vi "libdaq_gpio_read_bit.vi"(0 "error in (no error)":errorcluster, 1 "device_name":string, 2 "module_name":string, 4 "ioIndex":u8) -> (14 "error out":errorcluster, 15 "device_name":string, 16 "module_name":string, 18 "BitVal":bool=TRUE)   [LabVIEW 2010, in "libdaqVI.lvlib"]
doc: "读取一个输入IO的状态，对一个配置为OUT模式的IO执行读取操作，将会是该IO的输出电压，对一个配置为AF模式的IO执行读取操作，返回结果是不确定的"
uses:
  libdaqVI.lvlib
  dll/daqlib.dll
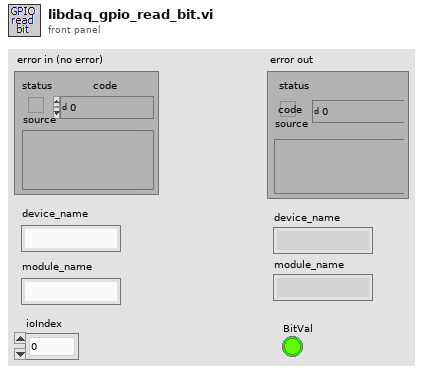
[diagram p1: front panel]
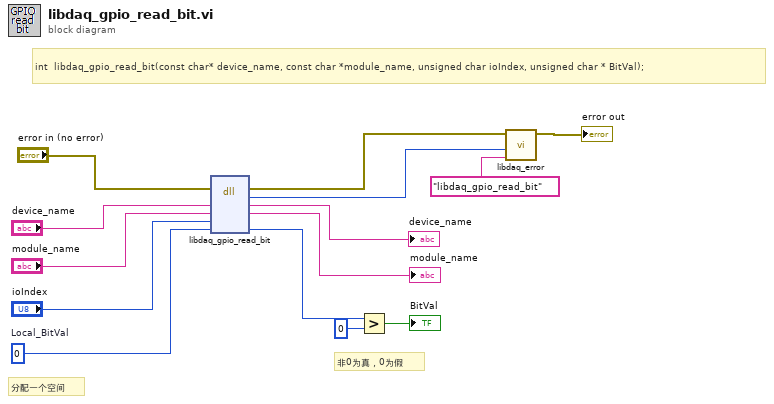
[diagram p0: block diagram]
diagram:
  w4 = u8 0  # Local_BitVal
  # "非0为真，0为假"
  # "分配一个空间"
  # "int  libdaq_gpio_read_bit(const char* device_name, const char *module_name, unsigned char ioIndex, unsigned char * BitVal);"
  n1 = dll-call lib="E:/Product/Example/DAQ-USB3212/Labview/labview_2010/libdaqVI/dll/daqlib.dll" fn="libdaq_gpio_read_bit"(error in="error in (no error)", "device_name"="device_name", "module_name"="module_name", "ioIndex"="ioIndex", "BitVal"=w4) -> (error out=w8:errorcluster, "return type"=w6:i32, "device_name"=→"device_name":string, "module_name"=→"module_name":string, "BitVal"=w3:u8)  [unwired: 3 in, 1 out]
  n2 = Greater?(x=w3, y=u8 0) -> (0:→"BitVal":bool)
  n3 = call "libdaq_error.vi"("error source"="libdaq_gpio_read_bit", "error code"=w6, "错误输入（无错误）"=w8) -> ("错误输出"=→"error out":errorcluster)  [unwired: 8 in]
